vi "enumerateStaticDependencies.vi"(8 "error in (no error)":errorcluster, 11 "Measurement.Free":refnum<class "Measurement.Free.lvclass">) -> (0 "error out":errorcluster, 2 "Static Dependencies":refnum<class "Dependency.lvclass">[](array[class]), 3 "Measurement.Free out":refnum<class "Measurement.Free.lvclass">)   [LabVIEW 2017, in "Measurement.Free.lvclass"]
doc: "JKI State Machine Objects (SMO) 1.1.0.20\nJKI - JKI\nCopyright (c) 2016, JKI"
uses:
  Measurement.Free.lvclass
  <vilib>/JKI/JKI SMO/Dependency/Dependency.lvclass
  SMU/SMU.lvclass
  D:/Program Files (x86)/National Instruments/LabVIEW 2017/vi.lib/JKI/JKI SMO/SMO/SMO.lvclass
  Typedefs/Dependencies--Cluster.ctl
  LIA/LIA.lvclass
  OPM/OPM.lvclass
  OPA/OPA.lvclass
  Device/Device.lvclass
  Measurement/Measurement.lvclass
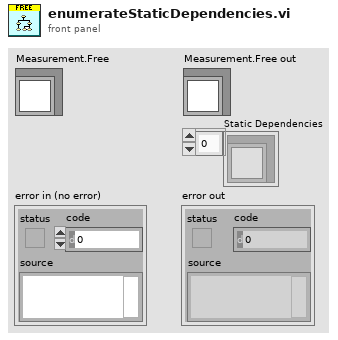
[diagram p1: front panel]
types:
  T1 = typedef "Measurement.Free.lvclass/Dependencies--Cluster.ctl" = cluster{"SMU":refnum<class "SMU.lvclass">, "LIA":refnum<class "LIA.lvclass">, "OPM":refnum<class "OPM.lvclass">, "OPA":refnum<class "OPA.lvclass">}
  T2 = typedef "Measurement.Free.lvclass/Configuration--Cluster.ctl" = cluster{"Measurement.Type":enum16{"Free", "I/V Curve", "Wavelength sweeping", "Photocurrent mapping"}, "Hardware":T3}
  T3 = typedef "Measurement.Free.lvclass/Configuration.Hardware--Cluster.ctl" = cluster{"SMU":T4, "LIA":T6, "OPM":T8, "OPA":T10}
  T4 = typedef "Measurement.lvclass/Configuration.SMU--Cluster.ctl" = cluster{"Enable":bool, "SMU Model":string, "Configuration":T5}
  T5 = typedef "SMU.lvclass/Configuration--Cluster.ctl" = cluster{"VISA Resource":string, "Channel":string}
  T6 = typedef "Measurement.lvclass/Configuration.LIA--Cluster.ctl" = cluster{"Enable":bool, "LIA Model":string, "Configuration":T7}
  T7 = typedef "LIA.lvclass/Configuration--Cluster.ctl" = cluster{"VISA Resource":string}
  T8 = typedef "Measurement.lvclass/Configuration.OPM--Cluster.ctl" = cluster{"Enable":bool, "OPM Model":string, "Configuration":T9}
  T9 = typedef "OPM.lvclass/Configuration--Cluster.ctl" = cluster{"VISA Resource":string}
  T10 = typedef "Measurement.lvclass/Configuration.OPA--Cluster.ctl" = cluster{"Enable":bool, "OPA Model":string, "Configuration":T11}
  T11 = typedef "OPA.lvclass/Configuration--Cluster.ctl" = cluster{"Serial Number":string}
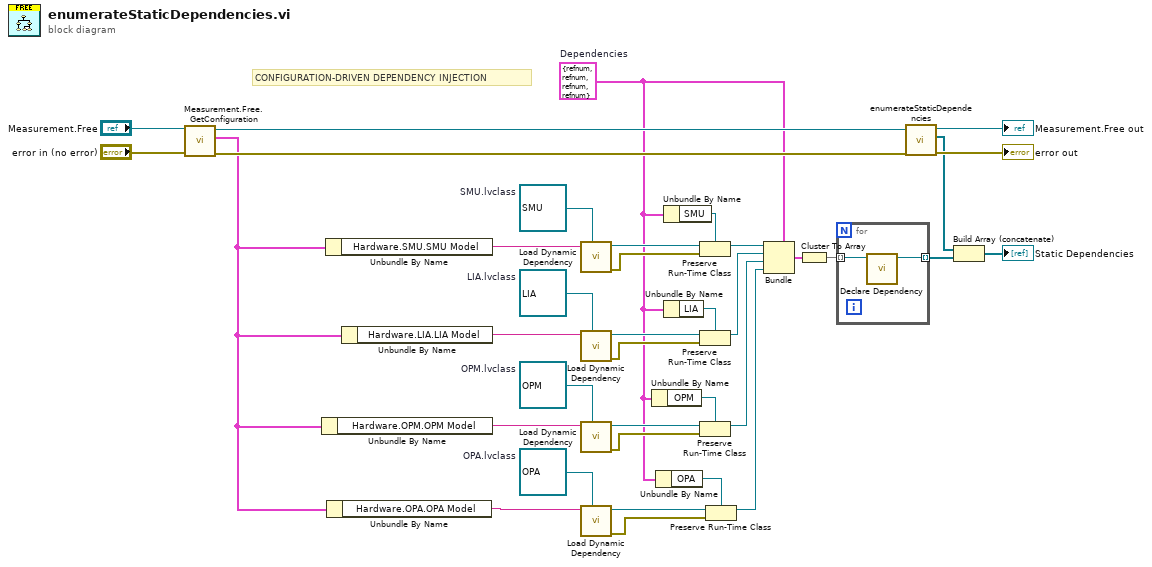
[diagram p0: block diagram]
diagram:
  w2 = refnum<class "OPA.lvclass"> refnum  # OPA.lvclass
  w13 = refnum<class "OPM.lvclass"> refnum  # OPM.lvclass
  w20 = refnum<class "LIA.lvclass"> refnum  # LIA.lvclass
  w3 = T1 {"SMU"=refnum, "LIA"=refnum, "OPM"=refnum, "OPA"=refnum}  # Dependencies
  w30 = refnum<class "SMU.lvclass"> refnum  # SMU.lvclass
  # "CONFIGURATION-DRIVEN DEPENDENCY INJECTION"
  n1 = call "Measurement.Free.GetConfiguration.vi"("error in (no error)"="error in (no error)", "Measurement.Free"="Measurement.Free") -> ("error out"=w22:errorcluster, "Configuration"=w8:T2, "Measurement.Free out"=w23:refnum<class "Measurement.Free.lvclass">)  [unwired: 7 in]
  n2 = Unbundle By Name(w8) -> ("Hardware.OPM.OPM Model"=w14:string)
  n3 = Unbundle By Name(w8) -> ("Hardware.SMU.SMU Model"=w31:string)
  n4 = Unbundle By Name(w8) -> ("Hardware.OPA.OPA Model"=w5:string)
  n5 = Unbundle By Name(w8) -> ("Hardware.LIA.LIA Model"=w15:string)
  n6 = call "Load Dynamic Dependency.vi"("SMO in"=w30, "Class Name"=w31) -> ("error out"=w27:errorcluster, "SMO out"=w28:refnum<class "SMU.lvclass">)  [unwired: 8 in]
  n7 = call "Load Dynamic Dependency.vi"("SMO in"=w20, "Class Name"=w15) -> ("error out"=w17:errorcluster, "SMO out"=w18:refnum<class "LIA.lvclass">)  [unwired: 8 in]
  n8 = call "Load Dynamic Dependency.vi"("SMO in"=w13, "Class Name"=w14) -> ("error out"=w11:errorcluster, "SMO out"=w12:refnum<class "OPM.lvclass">)  [unwired: 8 in]
  n9 = call "Load Dynamic Dependency.vi"("SMO in"=w2, "Class Name"=w5) -> ("error out"=w7:errorcluster, "SMO out"=w6:refnum<class "OPA.lvclass">)  [unwired: 8 in]
  n10 = Unbundle By Name(w3) -> ("OPM"=w10:refnum<class "OPM.lvclass">)
  n11 = Unbundle By Name(w3) -> ("OPA"=w4:refnum<class "OPA.lvclass">)
  n12 = Unbundle By Name(w3) -> ("SMU"=w29:refnum<class "SMU.lvclass">)
  n13 = Unbundle By Name(w3) -> ("LIA"=w19:refnum<class "LIA.lvclass">)
  n14 = Preserve Run-Time Class(object in=w28, error in=w27, 2:w29) -> (object out=w26:refnum<class "SMU.lvclass">)  [unwired: 1 out]
  n15 = Preserve Run-Time Class(object in=w18, error in=w17, 2:w19) -> (object out=w16:refnum<class "LIA.lvclass">)  [unwired: 1 out]
  n16 = Preserve Run-Time Class(object in=w12, error in=w11, 2:w10) -> (object out=w9:refnum<class "OPM.lvclass">)  [unwired: 1 out]
  n17 = Preserve Run-Time Class(object in=w6, error in=w7, 2:w4) -> (object out=w1:refnum<class "OPA.lvclass">)  [unwired: 1 out]
  n18 = Bundle(cluster=w3, "SMU"=w26, "LIA"=w16, "OPM"=w9, "OPA"=w1) -> (w25:T1)
  n19 = Cluster To Array(cluster=w25) -> (array=w24:refnum<class "Device.lvclass">[])
  n20 = for {
    tunnel: [w39] -> w35 mode=indexing
    tunnel: w24 -> [w38] mode=indexing
    n21 = call <vilib>:"Declare Dependency.vi"("Type"=w38) -> ("Dependency out"=w39:refnum<class "Dependency.lvclass">)  [unwired: 9 in, 1 out]
  }
  n22 = call-parent "enumerateStaticDependencies.vi"("error in (no error)"=w22, "SMO"=w23) -> ("error out"=→"error out":errorcluster, "Static Dependencies"=w34:refnum<class "Dependency.lvclass">[], "SMO out"=→"Measurement.Free out":refnum<class "Measurement.Free.lvclass">)  [unwired: 7 in]
  n23 = Build Array (concatenate)(w34, w35) -> (→"Static Dependencies":refnum<class "Dependency.lvclass">[])
